vi "playsound.vi"(8 "Volume":dbl=2.0, 9 "Mode":enum16{"Cue", "Success", "Failure", "Abort"}(ring), 10 "#S":dbl=5000.0, 11 "Fs":dbl=5000.0) -> ()   [LabVIEW 2011]
doc: "Opens a file and starts playing it immediately."
uses:
  <vilib>/sound2/lvsound2.llb/Sampling Mode.ctl
  <vilib>/sound2/lvsound2.llb/Sound Output Write (DBL Single).vi
  <vilib>/measure/NI_MABase.lvlib
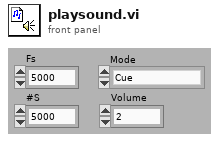
[diagram p1: front panel]
types:
  T1 = typedef "Sampling Mode.ctl" = i32
  T2 = typedef "Sound Output Task ID.ctl" = u32
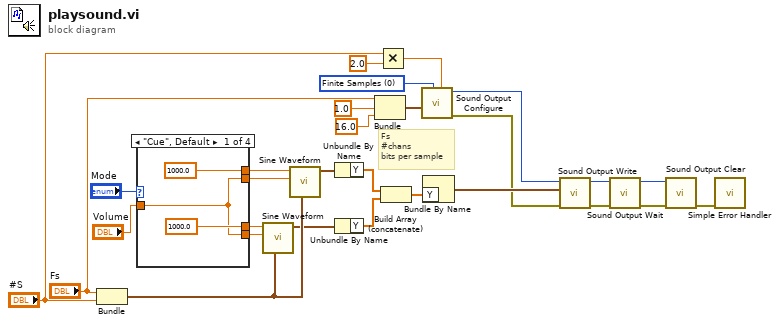
[diagram p0: block diagram]
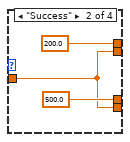
[diagram p2: hidden frame]
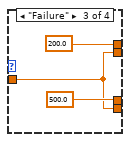
[diagram p3: hidden frame]
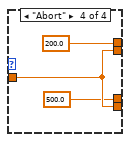
[diagram p4: hidden frame]
diagram:
  w28 = T1 0 items=["Finite Samples", "Continuous Samples"] ("sample mode")
  # "Fs\n#chans\nbits per sample"
  n1 = Bundle("Fs"="Fs", "#S"="#S") -> (w14:cluster{"Fs":dbl, "#S":dbl})  [unwired: 1 in]
  n2 = case shown="\"Cue\", Default" "Mode" {
    tunnel: [w29 w32 w35 w40] -> w27
    tunnel: [1000.0 ("frequency") 500.0 ("frequency") 500.0 ("frequency") 500.0 ("frequency")] -> w26
    tunnel: [1000.0 ("frequency") 200.0 ("frequency") 200.0 ("frequency") 200.0 ("frequency")] -> w16
    tunnel: [w29 w32 w35 w40] -> w15
    tunnel: "Volume" -> [w29 w32 w35 w40]
    frame "Cue", Default {
    }
    frame "Success" {
    }
    frame "Failure" {
    }
    frame "Abort" {
    }
  }
  n3 = call <vilib>:"Sine Waveform.vi"("sampling info"=w14, "amplitude"=w27, "frequency"=w26) -> ("signal out"=w12:waveform(dbl))  [unwired: 7 in, 1 out]
  n4 = call <vilib>:"Sine Waveform.vi"("sampling info"=w14, "amplitude"=w15, "frequency"=w16) -> ("signal out"=w13:waveform(dbl))  [unwired: 7 in, 1 out]
  n5 = Unbundle By Name(w13) -> ("Y"=w11:dbl[])
  n6 = Unbundle By Name(w12) -> ("Y"=w10:dbl[])
  n7 = Bundle("Fs"="Fs", 1.0, 16.0) -> (w23:cluster{"Fs":dbl, dbl, dbl})  [unwired: 1 in]
  n8 = Multiply(x="#S", y=2.0) -> (x*y=w7:dbl)
  n9 = Build Array (concatenate)(w11, w10) -> (w6:dbl[])
  n10 = call <vilib>:"Sound Output Configure.vi"("number of samples/ch"=w7, "sample mode"=w28, "sound format"=w23) -> ("error out"=w5:errorcluster, "task ID"=w17:T2)  [unwired: 7 in]
  n11 = Bundle By Name("Y"=w6) -> (w9:waveform(dbl))  [unwired: 1 in]
  n12 = call-poly <vilib>:"Sound Output Write.vi"("error in (no error)"=w5, "data"=w9, "task ID"=w17) -> ("error out"=w20:errorcluster, "task ID out"=w22:T2)  [unwired: 7 in]
  n13 = call <vilib>:"Sound Output Wait.vi"("error in (no error)"=w20, "task ID"=w22) -> ("error out"=w19:errorcluster, "task ID out"=w21:T2)  [unwired: 8 in]
  n14 = call <vilib>:"Sound Output Clear.vi"("error in (no error)"=w19, "task ID"=w21) -> ("error out"=w18:errorcluster)  [unwired: 9 in]
  n15 = call <vilib>:"Simple Error Handler.vi"("error in (no error)"=w18) -> ()  [unwired: 4 in, 5 out]
